vi "PRIME Detector Wait for Command to Complete original.vi"(8 "error in (no error)":errorcluster, 9 "Exp Time":dbl=60.0, 10 "timeout (120s)":dbl=120.0, 11 "connection ID":refnum<k5>) -> (0 "error out":errorcluster, 2 "Status":T1, 3 "connection ID out":refnum<k5>)   [LabVIEW 2021]
uses:
  PRIME Detector cluster Status.ctl
  PRIME Detector.lvclass
panel:
  out "Time Remaining":dbl(knob) scale=-1.0..10.0
  out "Command":string
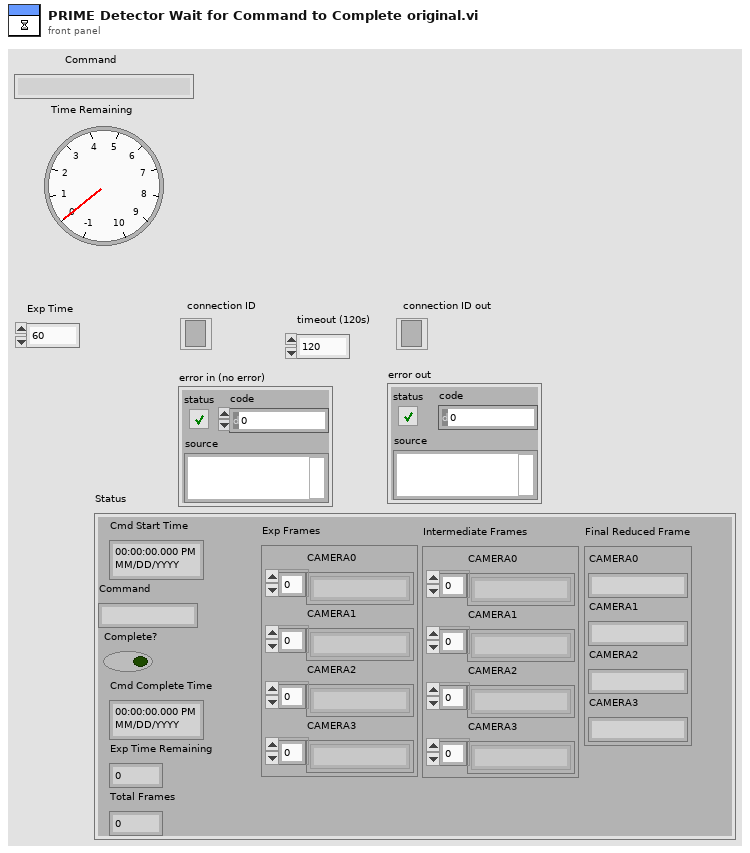
[diagram p1: front panel]
types:
  T1 = typedef "PRIME Detector cluster Status.ctl" = cluster{"Cmd Start Time":timestamp, "Command":string, "Complete?":bool, "Cmd Complete Time":timestamp, "Exp Time Remaining":dbl, "Total Frames":i32, "Exp Frames":cluster{"CAMERA0":string[], "CAMERA1":string[], "CAMERA2":string[], "CAMERA3":string[]}, "Intermediate Frames":cluster{"CAMERA0":string[], "CAMERA1":string[], "CAMERA2":string[], "CAMERA3":string[]}, "Final Reduced Frame":cluster{"CAMERA0":string, "CAMERA1":string, "CAMERA2":string, "CAMERA3":string}}
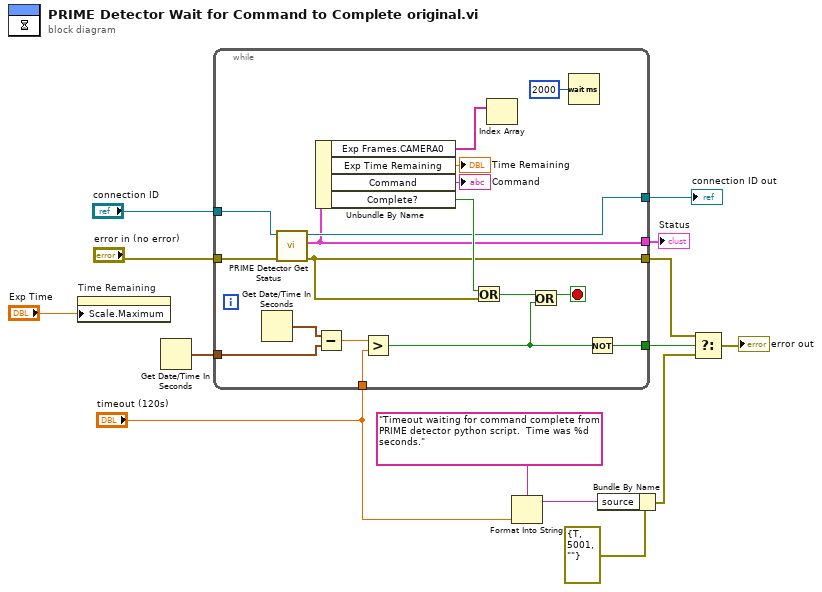
[diagram p0: block diagram]
diagram:
  n1 = property on="Time Remaining" class="Knob (strict)"("Scale.Maximum"="Exp Time") -> ()  [unwired: 2 in, 2 out]
  n2 = Get Date/Time In Seconds() -> (seconds since 1Jan1904=w12:timestamp)
  n3 = while {
    tunnel: "error in (no error)" -> [w32]
    tunnel: "connection ID" -> [w31]
    tunnel: [w28] -> w7
    tunnel: w12 -> [w25]
    tunnel: "timeout (120s)" -> [w23]
    tunnel: [w20] -> w10
    tunnel: [w19] -> w9
    tunnel: [w16] -> w8
    stop <- w18 stop-if-true
    n4 = Get Date/Time In Seconds() -> (seconds since 1Jan1904=w26:timestamp)
    n5 = call "PRIME Detector Get Status.vi"("error in (no error)"=w32, "connection ID"=w31) -> ("error out"=w28:errorcluster, "Status"=w19:T1, "connection ID out"=w20:refnum<k5>)  [unwired: 6 in, 1 out]
    n6 = Unbundle By Name(w19) -> ("Exp Frames.CAMERA0"=w15:string[], "Exp Time Remaining"=→"Time Remaining":dbl, "Command"=→"Command":string, "Complete?"=w30:bool)
    n7 = Subtract(x=w26, y=w25) -> (x-y=w24:dbl)
    n8 = Greater?(x=w24, y=w23) -> (0:w17:bool)
    n9 = Or(x=w30, y=w28) -> (x .or. y?=w29:bool)
    n10 = Index Array(array=w15) -> ()  [unwired: 1 in, 1 out]
    n11 = Or(x=w29, y=w17) -> (x .or. y?=w18:bool)
    n12 = Wait (ms)(milliseconds to wait=u32 2000 ("millisecond multiple")) -> ()  [unwired: 1 out]
    n13 = Not(x=w17) -> (.not. x?=w16:bool)
  }
  "connection ID out" <- w10
  "Status" <- w9
  n14 = Format Into String(format string="Timeout waiting for command complete from PRIME detector python script.  Time was %d seconds." ("source"), "timeout (120s)") -> (resulting string=w2:string)  [unwired: 2 in, 1 out]
  n15 = Bundle By Name(cluster=errorcluster {"status"=TRUE, "code"=5001, "source"=""} ("f"), "source"=w2) -> (w1:errorcluster)
  n16 = Select(t=w7, s=w8, f=w1) -> (s? t:f=→"error out":errorcluster)
